vi "RLC 공진주파수 병렬회로 실습.vi"() -> ()   [LabVIEW 2013]
panel:
  out "min Freq [Hz]":i32
  out "min Freq [Hz]":i32
  in  "정지":bool
  out "It min [mA]":dbl
  out "min ILC [mA]":dbl
  out "XY 그래프":cluster{i32[], dbl[]}[](graph)
  in  "C [uF]":dbl(slide) scale=0.0..0.2
  in  "L [mH]":dbl(slide) scale=0.0..100.0
  in  "R":dbl(slide) scale=0.0..1000.0
  in  "Vs":dbl(slide) scale=0.0..10.0
  # "1. L을 조절하여서 공진주파수를 5kHz를 만들고 싶다.\n이때 L의 값은? (단, Vs = 1, R=470, C=0.15)\n\n 답 : 6.754 [mH]\n\n 2. L을 조절하면서 주파수의 변동은 어떠한 식으로 나타나는가?\n\n 답 : 주파수가 처음에는 크게 줄어들다가, 점점 작게 줄어든다."
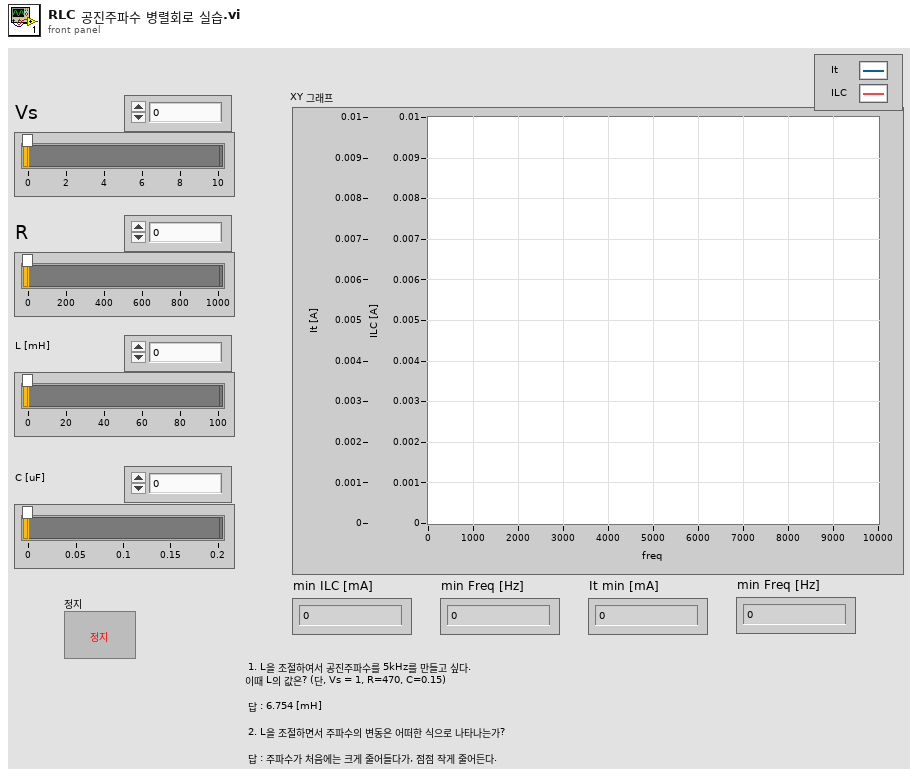
[diagram p1: front panel]
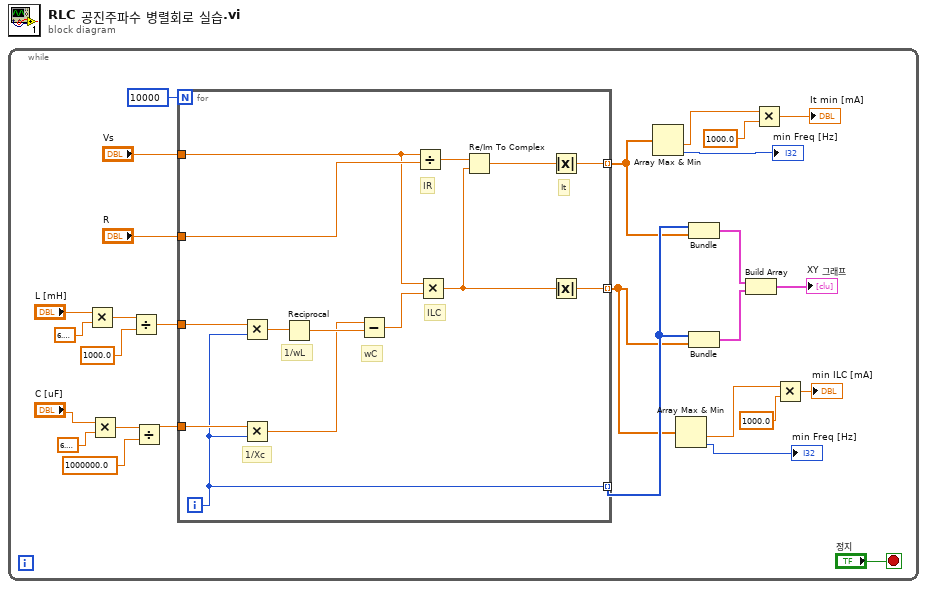
[diagram p0: block diagram]
diagram:
  n1 = while {
    stop <- "정지" stop-if-true
    n2 = Multiply(x="L [mH]", y=6.283185307179586) -> (x*y=w25:dbl)
    n3 = Multiply(x="C [uF]", y=6.283185307179586) -> (x*y=w20:dbl)
    n4 = Divide(x=w25, y=1000.0) -> (x/y=w17:dbl)
    n5 = Divide(x=w20, y=1000000.0) -> (x/y=w18:dbl)
    n6 = for {
      N: 10000 -> [_]
      tunnel: w18 -> [w42]
      tunnel: w17 -> [w41]
      tunnel: "Vs" -> [w36]
      tunnel: "R" -> [w37]
      tunnel: [w31] -> w14 mode=indexing
      tunnel: [w30] -> w13 mode=indexing
      tunnel: [w29] -> w12 mode=indexing
      i -> [w31]
      # "It"
      # "ILC"
      # "IR"
      # "wC"
      # "1/Xc"
      # "1/wL"
      n7 = Multiply(x=w41, y=w31) -> (x*y=w40:dbl)
      n8 = Multiply(x=w42, y=w31) -> (x*y=w38:dbl)
      n9 = Reciprocal(x=w40) -> (1/x=w39:dbl)
      n10 = Subtract(x=w38, y=w39) -> (x-y=w35:dbl)
      n11 = Divide(x=w36, y=w37) -> (x/y=w34:dbl)
      n12 = Multiply(x=w36, y=w35) -> (x*y=w32:dbl)
      n13 = Re/Im To Complex(1:w32, 2:w34) -> (0:w33:cdb)
      n14 = Absolute Value(x=w33) -> (abs(x)=w29:dbl)
      n15 = Absolute Value(x=w32) -> (abs(x)=w30:dbl)
    }
    n16 = Array Max & Min(array=w12) -> (min value=w11:dbl, min index (indices)=→"min Freq [Hz]":i32)  [unwired: 2 out]
    n17 = Array Max & Min(array=w13) -> (min value=w6:dbl, min index (indices)=→"min Freq [Hz]":i32)  [unwired: 2 out]
    n18 = Bundle(w14, w12) -> (w3:cluster{i32[], dbl[]})  [unwired: 1 in]
    n19 = Bundle(w14, w13) -> (w2:cluster{i32[], dbl[]})  [unwired: 1 in]
    n20 = Build Array(w3, w2) -> (→"XY 그래프":cluster{i32[], dbl[]}[])
    n21 = Multiply(x=w11, y=1000.0) -> (x*y=→"It min [mA]":dbl)
    n22 = Multiply(x=w6, y=1000.0) -> (x*y=→"min ILC [mA]":dbl)
  }
